vi "VCS Get Position Must.vi"(8 "error in (no error)":errorcluster, 11 "axis in":cluster{"keyHandle":u32, "nodeId":u16}={"keyHandle"=0, "nodeId"=1}) -> (0 "error out":errorcluster, 2 "positionMust":i32, 3 "axis out":cluster{"keyHandle":u32, "nodeId":u16}={"keyHandle"=0, "nodeId"=1})   [LabVIEW 2019, in "maxonEPOS.lvlib"]
doc: "<B>VCS Get Position Must</B> reads the position demand value."
uses:
  Examples/maxonEPOS.lvlib
  Resources/EposCmd.dll
  Resources/EposCmd64.dll
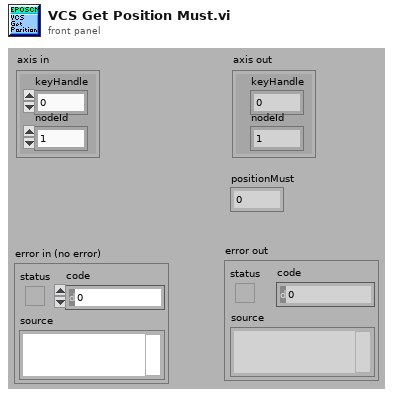
[diagram p1: front panel]
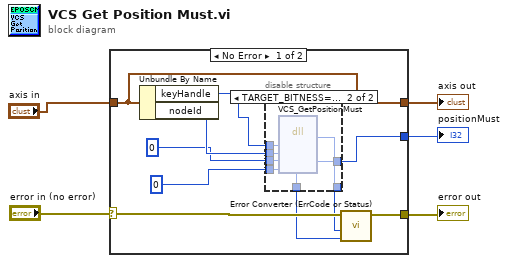
[diagram p0: block diagram]
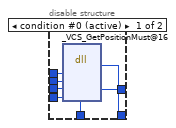
[diagram p2: hidden frame]
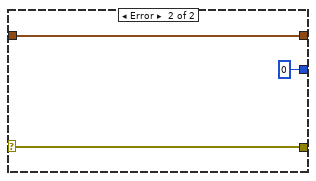
[diagram p3: hidden frame]
diagram:
  n1 = case shown="No Error" "error in (no error)" {
    selector: "error in (no error)" -> [w15 w30]
    tunnel: "axis in" -> [w10 w32]
    tunnel: [w10 w32] -> w3
    tunnel: [w9 w30] -> w2
    tunnel: [w8 0 ("pPositionMust")] -> w1
    frame No Error {
      n2 = Unbundle By Name(w10) -> ("keyHandle"=w13:u32, "nodeId"=w12:u16)
      n3 = disable-structure shown="TARGET_BITNESS==64" {
        disable-tunnel: [w22 w29] -> w14
        disable-tunnel: w13 -> [w21 w28]
        disable-tunnel: w12 -> [w20 w27]
        disable-tunnel: u32 0 ("pErrorCode") -> [w19 w26]
        disable-tunnel: [w18 w25] -> w8
        disable-tunnel: 0 ("pPositionMust") -> [w17 w24]
        disable-tunnel: [w16 w23] -> w6
        frame condition #0 (active) {
          n4 = dll-call lib="C:/workspace/project/scancon/sw/SSI_Tool/InstrumentsInterfaces/Motordriver/maxon EPOS/Resources/EposCmd.*" fn="_VCS_GetPositionMust@16"("KeyHandle"=w21, "NodeId"=w20, "pPositionMust"=w17, "pErrorCode"=w19) -> (w16:i32, "pPositionMust"=w18:i32, "pErrorCode"=w22:u32)  [unwired: 5 in, 2 out]
        }
        frame condition #1 {
          n5 = dll-call lib="C:/setup/Resources/EposCmd64.*" fn="VCS_GetPositionMust" ("EposCmd.dll:_VCS_GetPositionMust@16")("KeyHandle"=w28, "NodeId"=w27, "pPositionMust"=w24, "pErrorCode"=w26) -> ("Rückgabetyp"=w23:i32, "pPositionMust"=w25:i32, "pErrorCode"=w29:u32)  [unwired: 5 in, 2 out]
        }
      }
      n6 = call "Error Converter (ErrCode or Status).vi"("error code"=w14, "return type"=w6, "error in (no error)"=w15) -> ("error out"=w9:errorcluster)  [unwired: 7 in]
    }
    frame Error {
    }
  }
  "positionMust" <- w1
  "error out" <- w2
  "axis out" <- w3
